vi "HDPE Threshold and retain req particles.vi"(8 "error in (no error)":errorcluster, 9 "Buffer":i32, 10 "Color ranges":T2={"Color Mode "=0, "Red or Hue Range"={"Lower value"=202, "Upper value"=255}, "Green or Sat Range"={"Lower value"=144, "Upper value"=234}, "Blue or Luma or Val \nor Inten Range"={"Lower value"=7, "Upper value"=150}} {"Color Mode" items=["RGB", "HSL", "HSV", "HSI"]}, 11 "Refnum in":T1) -> (0 "error out":errorcluster, 3 "Image Out":T1)   [LabVIEW 2019]
uses:
  <vilib>/vision/Image Controls.llb/IMAQ Image.ctl
  Controls/Color Range cluster.ctl
  <vilib>/vision/NI_Vision_Development_Module.lvlib
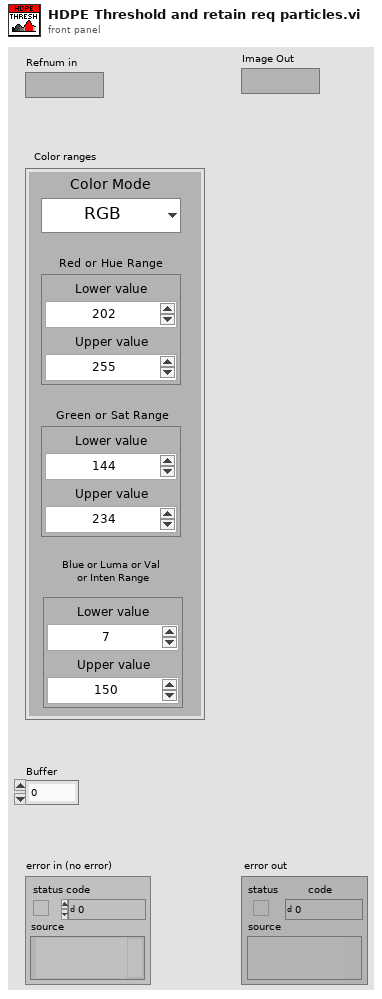
[diagram p1: front panel]
types:
  T1 = typedef "IMAQ Image.ctl" = refnum<image>
  T2 = typedef "Color Range cluster.ctl" = cluster{"Color Mode ":u16, "Red or Hue Range":cluster{"Lower value":i32, "Upper value":i32}, "Green or Sat Range":cluster{"Lower value":i32, "Upper value":i32}, "Blue or Luma or Val \nor Inten Range":cluster{"Lower value":i32, "Upper value":i32}}
  T3 = cluster{"histogram":u32[], "Minimal Value":sgl, "Maximal Value":sgl, "Starting Value":sgl, "Interval Width":sgl, "Mean Value":sgl, "Standard  Variation":sgl, "Area (pixels)":i32}
  T4 = typedef "Image Type" = u32
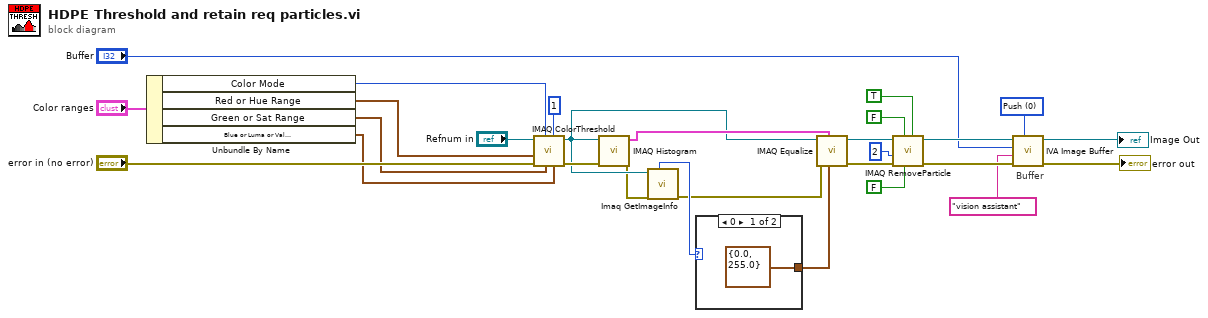
[diagram p0: block diagram]
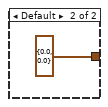
[diagram p2: hidden frame]
diagram:
  w11 = u16 0 items=["Push", "Pop", "Reset"] ("Function")
  # "Buffer"
  n1 = Unbundle By Name("Color ranges") -> ("Color Mode"=w3:u16, "Red or Hue Range"=w6:cluster{"Lower value":i32, "Upper value":i32}, "Green or Sat Range"=w5:cluster{"Lower value":i32, "Upper value":i32}, "Blue or Luma or Val \nor Inten Range"=w4:cluster{"Lower value":i32, "Upper value":i32})
  n2 = call "IMAQ ColorThreshold"("Blue or Luma or Val or Inten Range"=w4, "Replace Value"=1, "Green or Sat Range"=w5, "Color Mode"=w3, "error in (no error)"="error in (no error)", "Red or Hue Range"=w6, "Image Src"="Refnum in") -> ("error out"=w26:errorcluster, "Image Dst Out"=w22:T1)  [unwired: 1 in, 2 out]
  n3 = call "IMAQ Histogram"("error in (no error)"=w26, "Image"=w22) -> ("error out"=w21:errorcluster, "Histogram Report"=w24:T3)  [unwired: 3 in, 5 out]
  n4 = call "Imaq GetImageInfo"("error in (no error)"=w21, "Image"=w22) -> ("error out"=w20:errorcluster, "Image Type"=w23:T4)  [unwired: 8 out]
  n5 = case shown="0" w23 {
    tunnel: [cluster{"Minimum":sgl, "Maximum":sgl} {"Minimum"=0.0, "Maximum"=255.0} ("Range") cluster{"Minimum":sgl, "Maximum":sgl} {"Minimum"=0.0, "Maximum"=0.0} ("Range")] -> w19
    frame 0 {
    }
    frame Default {
    }
  }
  n6 = call "IMAQ Equalize"("Range"=w19, "Histogram Report"=w24, "error in (no error)"=w20, "Image Src"=w22) -> ("error out"=w25:errorcluster, "Image Dst Out"=w14:T1)  [unwired: 2 in, 4 out]
  n7 = call "IMAQ RemoveParticle"("Connectivity 4/8 (8)"=TRUE, "Low Pass/High Pass (Low)"=FALSE, "Square/Hexa (Square)"=FALSE, "error in (no error)"=w25, "Number of Erosion"=2, "Image Src"=w14) -> ("error out"=w13:errorcluster, "Image Dst Out"=w12:T1)  [unwired: 1 in, 3 out]
  n8 = call <vilib>:"IVA Image Buffer.vi"("Function"=w11, "error in (no error)"=w13, "Prefix"="vision assistant", "Buffer #"="Buffer", "Image In"=w12) -> ("error out"=→"error out":errorcluster, "Image Out"=→"Image Out":T1)  [unwired: 5 out]
